vi "SysID Tracking.vi"(6 "PID Cluster":T4={"L1 to L4 PID Cluster"={"L1 PID Gains"={"Kp"=0.005, "Kd"=0.5, "Ki"=0.0005}, "L2 PID Gains"={"Kp"=0.01, "Kd"=1.0, "Ki"=0.005}, "L3 PID Gains"={"Kp"=0.05, "Kd"=1.0, "Ki"=0.0005}, "L4 PID Gains"={"Kp"=0.1, "Kd"=0.1, "Ki"=0.0005}}, "Stage PID Cluster"={"Stage Z PID"={"Kp"=0.0005, "Kd"=0.001, "Ki"=0.0}, "Stage Y PID"={"Kp"=0.0003, "Kd"=0.01, "Ki"=0.0}, "Stage X PID"={"Kp"=0.0003, "Kd"=0.01, "Ki"=0.0}}, "OCT Z PID Gains"={"Kp"=0.0003, "Kd"=0.0001, "Ki"=0.01}}, 7 "Input RY Signals":T1, 8 "error in":errorcluster, 9 "Offset Home 2 RCM":dbl[](array[numeric])=[0.0, 0.0, 0.0, 0.0], 10 "Prev Posit Cmd":T3={"Prev L1 to L4 Posit"=[-0.5319, -0.035669172703475985, -2.0566170657346783, 0.9099264705882353], "Prev Stage Posit"=[6.002553885707208, 5.996566124542428, 5.995469940427586], "Prev OCT Z Posit"=-0.0}, 11 "FPGA VI Reference In":refnum<k20>) -> (0 "error out":errorcluster, 2 "Last Posit Cmd":T2={"Last L1 to L4 Posit"=[0.0, 0.0, 0.0, 0.0], "Last Stage Posit"=[6.0, 6.0, 6.0], "Last OCT Z Posit"=0.0}, 3 "FPGA VI Reference Out":refnum<k20>, 5 "Output RY Signals":T1)   [LabVIEW 2016]
uses:
  <vilib>/Platform/TimedLoop/XDataNode/timing_clust.ctl
  <vilib>/Platform/TimedLoop/XDataNode/nitl_modes.ctl
  <vilib>/Platform/TimedLoop/XDataNode/wakeup.ctl
  Global Variables.vi
  <vilib>/Platform/TimedLoop/XDataNode/XDataNode.xnode
  <vilib>/Platform/TimedLoop/XDataNode/XDNodeRunTimeDep.lvlib
  Library/KevinLibraryAll/labview/KevLib01.lvlib
panel:
  out "In Servo Loop":bool
  out "Loading Finished":bool
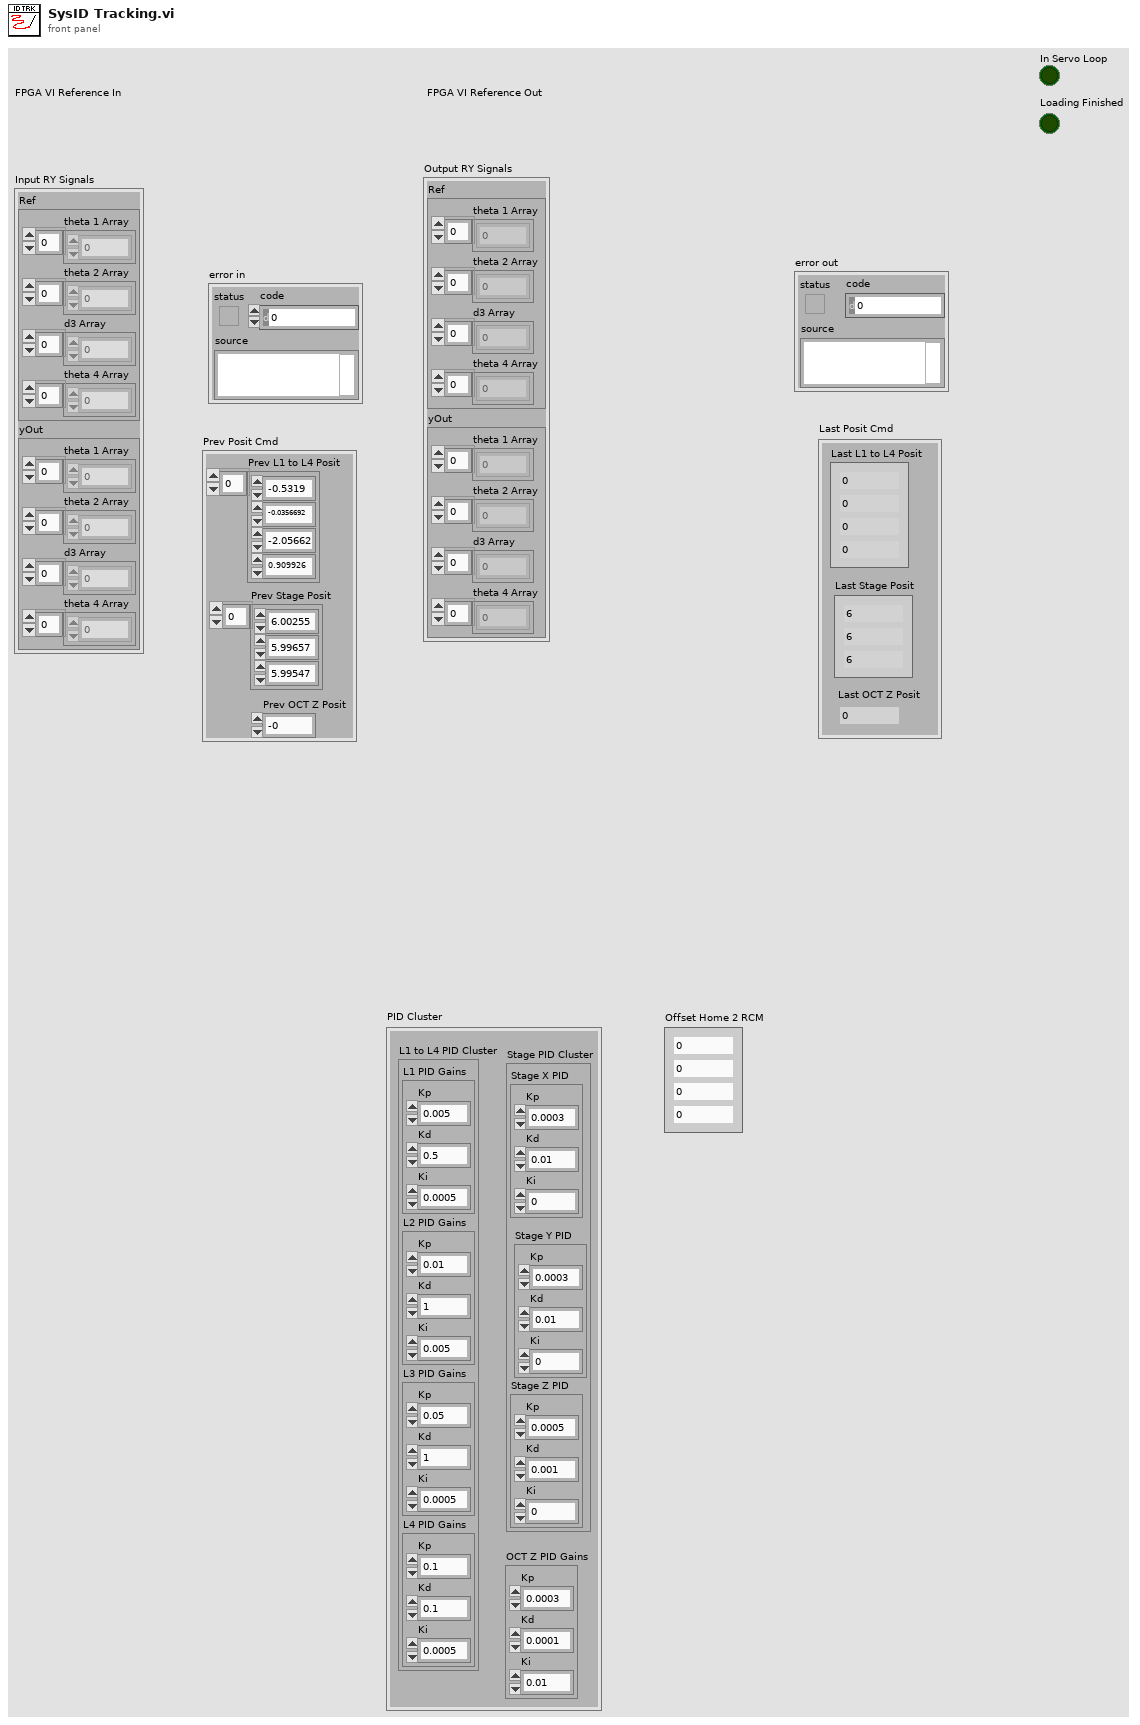
[diagram p1: front panel]
types:
  T1 = cluster{"Ref":cluster{"theta 1 Array":dbl[], "theta 2 Array":dbl[], "d3 Array":dbl[], "theta 4 Array":dbl[]}, "yOut":cluster{"theta 1 Array":dbl[], "theta 2 Array":dbl[], "d3 Array":dbl[], "theta 4 Array":dbl[]}}
  T2 = cluster{"Last L1 to L4 Posit":dbl[], "Last Stage Posit":dbl[], "Last OCT Z Posit":dbl}
  T3 = cluster{"Prev L1 to L4 Posit":dbl[], "Prev Stage Posit":dbl[], "Prev OCT Z Posit":dbl}
  T4 = cluster{"L1 to L4 PID Cluster":cluster{"L1 PID Gains":cluster{"Kp":dbl, "Kd":dbl, "Ki":dbl}, "L2 PID Gains":cluster{"Kp":dbl, "Kd":dbl, "Ki":dbl}, "L3 PID Gains":cluster{"Kp":dbl, "Kd":dbl, "Ki":dbl}, "L4 PID Gains":cluster{"Kp":dbl, "Kd":dbl, "Ki":dbl}}, "Stage PID Cluster":cluster{"Stage Z PID":cluster{"Kp":dbl, "Kd":dbl, "Ki":dbl}, "Stage Y PID":cluster{"Kp":dbl, "Kd":dbl, "Ki":dbl}, "Stage X PID":cluster{"Kp":dbl, "Kd":dbl, "Ki":dbl}}, "OCT Z PID Gains":cluster{"Kp":dbl, "Kd":dbl, "Ki":dbl}}
  T5 = cluster{"Stop Vacuum":bool, "Vacuum Force":i8, "Max Limit [mmHg]":dbl, "Slide in":i8, "Irrigation?":bool}
  T6 = typedef "XDNodeRunTimeDep.lvlib/timing_clust.ctl" = cluster{"Expected End [f-1]":u64, "Actual End [f-1]":u64, "Finished Late? [f-1]":bool, "Expected End [i-1]":u64, "Actual End [i-1]":u64, "Finished Late? [i-1]":bool, "Expected Start [i]":u64, "Actual Start [i]":u64, "Expected Start [f]":u64, "Actual Start [f]":u64, "Source Name":string, "Structure Name":string, "Period":i64, "Deadline":i64, "Offset":i64, "Start":i64, "Priority":i32, "Timeout":i32, "Mode":T7, "Wakeup Reason":T8, "Error":errorcluster, "Source Type":string, "Secondary Source Type":string, "Global End Time":u64, "Global Start Time":u64, "Frame Duration":u64, "Iteration Duration":u64, "Assigned CPU":i32, "I/O Scan Engine Mode":u32}
  T7 = typedef "XDNodeRunTimeDep.lvlib/nitl_modes.ctl" = enum32{"No Change", "Process missed periods, maintain original phase", "Discard missed periods, maintain original phase", "Process missed periods, ignore original phase", "Discard missed periods, ignore original phase"}
  T8 = typedef "XDNodeRunTimeDep.lvlib/wakeup.ctl" = enum32{"Normal", "Aborted", "Asynchronous wakeup", "Timing source error", "Timed loop error", "Timeout"}
  T9 = cluster{"L1 PID Gains":cluster{"Kp":dbl, "Kd":dbl, "Ki":dbl}, "L2 PID Gains":cluster{"Kp":dbl, "Kd":dbl, "Ki":dbl}, "L3 PID Gains":cluster{"Kp":dbl, "Kd":dbl, "Ki":dbl}, "L4 PID Gains":cluster{"Kp":dbl, "Kd":dbl, "Ki":dbl}}
  T10 = cluster{"Stage Z PID":cluster{"Kp":dbl, "Kd":dbl, "Ki":dbl}, "Stage Y PID":cluster{"Kp":dbl, "Kd":dbl, "Ki":dbl}, "Stage X PID":cluster{"Kp":dbl, "Kd":dbl, "Ki":dbl}}
  T11 = cluster{"Accurus button":bool[], "Accurus engaged?":bool, "Vacuum Force":i32, "Accurus Ch. A Vout":dbl, "Accurus Ch. B Vout":dbl, "Irrigation engaged?":bool}
  T12 = cluster{"theta 1 Array":dbl[], "theta 2 Array":dbl[], "d3 Array":dbl[], "theta 4 Array":dbl[]}
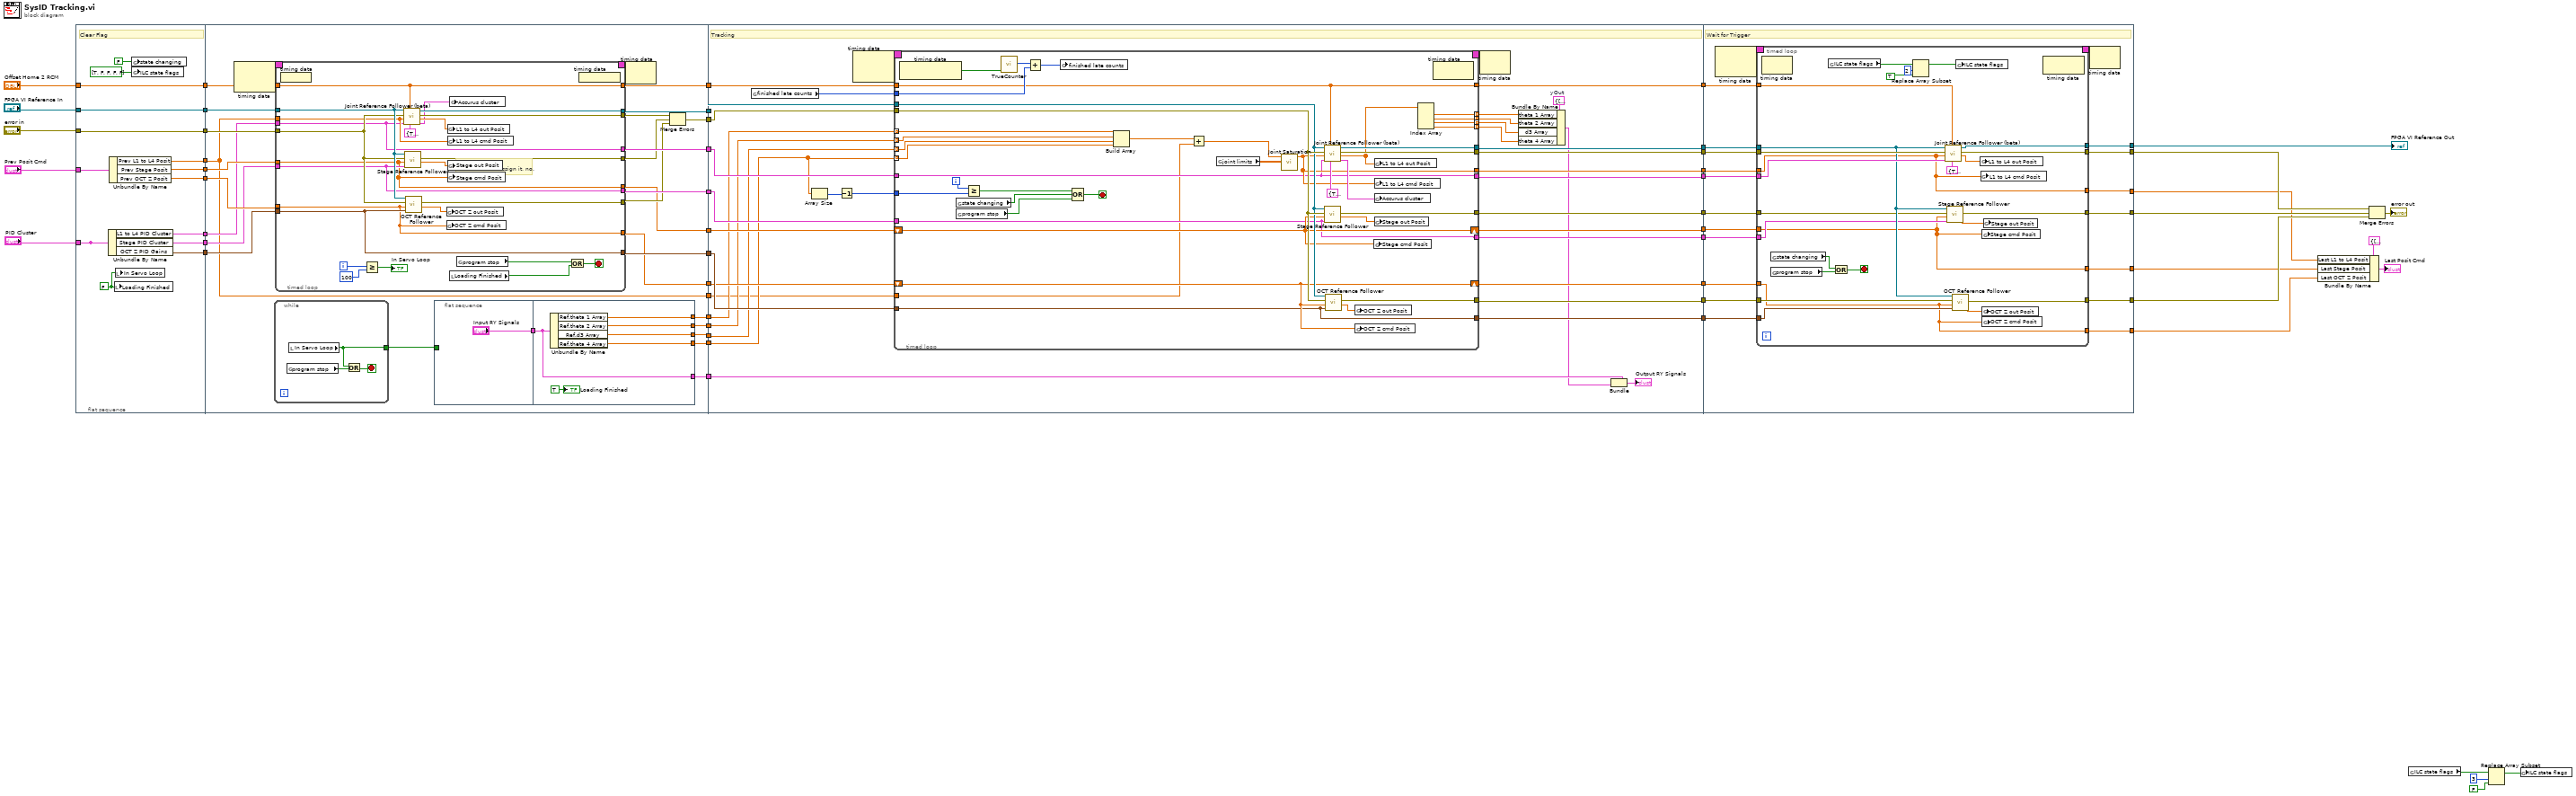
[diagram p0: block diagram]
diagram:
  n1 = flat-sequence {
    tunnel: [w67] -> w53
    tunnel: "FPGA VI Reference In" -> [w67]
    tunnel: "error in" -> [w66]
    tunnel: [w66] -> w51
    tunnel: "Prev Posit Cmd" -> [w65]
    tunnel: [w64] -> _
    tunnel: "PID Cluster" -> [w64]
    tunnel: [w63] -> w48
    tunnel: [w62] -> w47
    tunnel: [w61] -> w46
    tunnel: [w60] -> w45
    tunnel: [w59] -> w44
    tunnel: "Offset Home 2 RCM" -> [w59]
    tunnel: [w58] -> w39
    tunnel: [w56] -> w32
    tunnel: w53 -> [w96]
    tunnel: w51 -> [w95]
    tunnel: w48 -> [w94]
    tunnel: w47 -> [w93]
    tunnel: w46 -> [w92]
    tunnel: w45 -> [w91]
    tunnel: w44 -> [w90]
    tunnel: [w89] -> w42
    tunnel: [w88] -> w41
    tunnel: [w87] -> w40
    tunnel: w39 -> [w86]
    tunnel: [w85] -> w38
    tunnel: [w84] -> w37
    tunnel: [w83] -> w36
    tunnel: w32 -> [w68]
    tunnel: [w77] -> w31
    tunnel: [w76] -> w30
    tunnel: [w73] -> w25
    tunnel: [w72] -> w24
    tunnel: [w71] -> w23
    tunnel: [w70] -> w22
    tunnel: [w69] -> w21
    tunnel: [w68] -> w14
    tunnel: w42 -> [w169]
    tunnel: w41 -> [w155]
    tunnel: w40 -> [w168]
    tunnel: w38 -> [w166]
    tunnel: w37 -> [w165]
    tunnel: w36 -> [w164]
    tunnel: w31 -> [w157]
    tunnel: w30 -> [w156]
    tunnel: w25 -> [w140]
    tunnel: w24 -> [w151]
    tunnel: w23 -> [w150]
    tunnel: w22 -> [w149]
    tunnel: w21 -> [w148]
    tunnel: [w163] -> w13
    tunnel: [w162] -> w12
    tunnel: [w161] -> w11
    tunnel: [w160] -> w10
    tunnel: [w152] -> w9
    tunnel: [w159] -> w8
    tunnel: [w158] -> w7
    tunnel: [w142] -> w6
    tunnel: [w141] -> w5
    tunnel: [w139] -> w4
    tunnel: [w138] -> w3
    tunnel: w14 -> [w136]
    tunnel: w13 -> [w233]
    tunnel: w12 -> [w232]
    tunnel: w11 -> [w226]
    tunnel: w10 -> [w227]
    tunnel: w9 -> [w231]
    tunnel: w8 -> [w229]
    tunnel: w7 -> [w228]
    tunnel: w6 -> [w234]
    tunnel: w5 -> [w230]
    tunnel: w3 -> [w225]
    tunnel: w4 -> [w224]
    tunnel: [w223] -> w18
    tunnel: [w222] -> w19
    tunnel: [w221] -> w20
    tunnel: [w220] -> w1
    tunnel: [w219] -> w17
    tunnel: [w218] -> w16
    tunnel: [w217] -> w15
    frame #0 {
      w57 = FALSE ("Loading Finished")
      # "Clear Flag"
      n2 = Unbundle By Name(w64) -> ("L1 to L4 PID Cluster"=w60:T9, "Stage PID Cluster"=w58:T10, "OCT Z PID Gains"=w63:cluster{"Kp":dbl, "Kd":dbl, "Ki":dbl})
      n3 = Unbundle By Name(w65) -> ("Prev L1 to L4 Posit"=w56:dbl[], "Prev Stage Posit"=w62:dbl[], "Prev OCT Z Posit"=w61:dbl)
      n4 = local write "Loading Finished"(w57) -> ()
      n5 = local write "In Servo Loop"(w57) -> ()
      n6 = global write "Global Variables.vi" "state changing"(FALSE ("state changing")) -> ()
      n7 = global write "Global Variables.vi" "ILC state flags"(bool[] [TRUE, FALSE, FALSE, FALSE, FALSE]) -> ()
    }
    frame #1 {
      # "terminate loop\nwhen it. no. > assign it. no."
      n8 = node-c288() -> (w82:T6)  [unwired: 2 in]
      n9 = while {
        tunnel: [w97] -> w75
        stop <- w99 stop-if-true
        n10 = global read "Global Variables.vi" "program stop"() -> (w98:bool)
        n11 = local read "In Servo Loop"() -> (w97:bool)
        n12 = Or(x=w97, y=w98) -> (x .or. y?=w99:bool)
      }
      n13 = timed-loop {
        timing: w82 -> [_]
        timing-out: [_] -> w81
        tunnel: [w108] -> w77
        tunnel: [w107] -> w76
        tunnel: [w124] -> w89
        tunnel: [w123] -> w80
        tunnel: [w122] -> w79
        tunnel: [w121] -> w78
        tunnel: w96 -> [w120]
        tunnel: w95 -> [w119]
        tunnel: w94 -> [w116]
        tunnel: w68 -> [w118]
        tunnel: w93 -> [w108]
        tunnel: w92 -> [w107]
        tunnel: w91 -> [w114]
        tunnel: w90 -> [w117]
        tunnel: [w117] -> w88
        tunnel: w86 -> [w115]
        tunnel: [w116] -> w83
        tunnel: [w115] -> w84
        tunnel: [w114] -> w85
        i -> [w113]
        stop <- w130 stop-if-true
        n14 = node-c288 ("Output Node")() -> ()  [unwired: 1 in]
        n15 = Greater Or Equal?(x=w113, y=100) -> (x >= y?=→"In Servo Loop":bool)
        n16 = call "Joint Reference Follower (beta).vi"("Accurus Ctrl Cluster"=T5 {"Stop Vacuum"=TRUE, "Vacuum Force"=0, "Max Limit [mmHg]"=600.0, "Slide in"=0, "Irrigation?"=TRUE}, "Offset Home2RCM [deg/mm]"=w117, "PID Ctrl Cluster"=w114, "Ref Array [deg/mm]"=w118, "error in"=w119, "FPGA VI Reference In"=w120) -> ("Accurus Output Cluster"=w109:T11, "Output Posit Array [deg/mm]"=w127:dbl[], "error out"=w123:errorcluster, "FPGA VI Reference Out"=w124:refnum<k20>)  [unwired: 2 in]
        n17 = call "Stage Reference Follower.vi"("Stage PID Cluster"=w115, "Stage cmd Posit [mm]"=w108, "error in"=w119, "FPGA VI Reference In"=w120) -> ("Stage out Posit [mm]"=w126:dbl[], "error out"=w122:errorcluster)  [unwired: 5 in, 1 out]
        n18 = call "OCT Reference Follower.vi"("OCT Z PID Gains"=w116, "OCT  Z cmd Posit [mm]"=w107, "error in"=w119, "FPGA VI Reference In"=w120) -> ("OCT  Z out Posit [mm]"=w125:dbl, "error out"=w121:errorcluster)  [unwired: 5 in, 1 out]
        n19 = global write "Global Variables.vi" "OCT Z out Posit"(w125) -> ()
        n20 = global write "Global Variables.vi" "OCT Z cmd Posit"(w107) -> ()
        n21 = global write "Global Variables.vi" "L1 to L4 out Posit"(w127) -> ()
        n22 = global write "Global Variables.vi" "L1 to L4 cmd Posit"(w118) -> ()
        n23 = global write "Global Variables.vi" "Stage out Posit"(w126) -> ()
        n24 = global write "Global Variables.vi" "Stage cmd Posit"(w108) -> ()
        n25 = global write "Global Variables.vi" "Accurus cluster"(w109) -> ()
        n26 = local read "Loading Finished"() -> (w129:bool)
        n27 = global read "Global Variables.vi" "program stop"() -> (w128:bool)
        n28 = Or(x=w128, y=w129) -> (x .or. y?=w130:bool)
        n29 = node-c288() -> ()  [unwired: 1 out]
      }
      n30 = flat-sequence {
        tunnel: w75 -> [_]
        tunnel: ["Input RY Signals"] -> w74
        tunnel: w74 -> [w101]
        tunnel: [w105] -> w72
        tunnel: [w104] -> w71
        tunnel: [w103] -> w70
        tunnel: [w102] -> w69
        tunnel: [w101] -> w73
        frame #0 {
        }
        frame #1 {
          n31 = Unbundle By Name(w101) -> ("Ref.theta 1 Array"=w105:dbl[], "Ref.theta 2 Array"=w104:dbl[], "Ref.d3 Array"=w103:dbl[], "Ref.theta 4 Array"=w102:dbl[])
          "Loading Finished" <- TRUE ("Loading Finished")
        }
      }
      n32 = node-c288(w81) -> ()  [unwired: 1 out]
      n33 = Merge Errors(w80, w79, w78) -> (w87:errorcluster)
    }
    frame #2 {
      w147 = T12 {"theta 1 Array"=[], "theta 2 Array"=[], "d3 Array"=[], "theta 4 Array"=[]}  # yOut
      # "Tracking"
      n34 = global read "Global Variables.vi" "finished late counts"() -> (w167:u16)
      n35 = Array Size(array=w148) -> (size(s)=w154:i32)
      n36 = Decrement(x=w154) -> (x-1=w153:i32)
      n37 = node-c288() -> (w171:T6)  [unwired: 2 in]
      n38 = timed-loop {
        timing: w171 -> [_]
        timing-out: [_] -> w170
        tunnel: w151 -> [w189] mode=indexing
        tunnel: w150 -> [w188] mode=indexing
        tunnel: w149 -> [w187] mode=indexing
        tunnel: w169 -> [w209]
        tunnel: w155 -> [w178]
        tunnel: w168 -> [w210]
        tunnel: [w211] -> w163
        tunnel: w166 -> [w177]
        tunnel: w167 -> [w205]
        tunnel: w165 -> [w176]
        tunnel: w164 -> [w175]
        shift-right: [w202] -> w159
        shift-left: w157 -> [w202]
        shift-right: [w201] -> w158
        shift-left: w156 -> [w201]
        tunnel: [w200] -> w161
        tunnel: [w199] -> w160
        tunnel: [w198] -> w162
        tunnel: w153 -> [w195]
        tunnel: w148 -> [w186] mode=indexing
        tunnel: [w185] -> w152
        tunnel: [w182] -> w146 mode=indexing
        tunnel: [w181] -> w145 mode=indexing
        tunnel: [w180] -> w144 mode=indexing
        tunnel: [w179] -> w143 mode=indexing
        tunnel: [w178] -> w142
        tunnel: [w177] -> w141
        tunnel: [w176] -> w138
        tunnel: [w175] -> w139
        tunnel: w136 -> [w174]
        i -> [w190]
        stop <- w191 stop-if-true
        # "Hold Position if not Engaged"
        n39 = node-c288() -> (w208:bool)  [unwired: 1 in]
        n40 = global read "Global Variables.vi" "state changing"() -> (w193:bool)
        n41 = global read "Global Variables.vi" "program stop"() -> (w192:bool)
        n42 = Greater Or Equal?(x=w190, y=w195) -> (x >= y?=w194:bool)
        n43 = call "TrueCounter.vi"("True?"=w208) -> ("True Count"=w206:u16)  [unwired: 10 in]
        n44 = Add(x=w206, y=w205) -> (x+y=w207:u16)
        n45 = global write "Global Variables.vi" "finished late counts"(w207) -> ()
        n46 = Compound Arithmetic op=OR(w194, w193, w192) -> (w191:bool)
        n47 = Build Array(w189, w188, w187, w186) -> (w173:dbl[])
        n48 = Add(x=w173, y=w174) -> (x+y=w172:dbl[])
        n49 = global read "Global Variables.vi" "joint limits"() -> (w184:dbl[][])
        n50 = call "Joint Saturation.vi"("Joint Bounds [Deg/mm]"=w184, "Ref Array [Deg/mm]"=w172) -> ("Sat Ref Array [Deg/mm]"=w185:dbl[])  [unwired: 9 in]
        n51 = call "Joint Reference Follower (beta).vi"("Accurus Ctrl Cluster"=T5 {"Stop Vacuum"=TRUE, "Vacuum Force"=0, "Max Limit [mmHg]"=600.0, "Slide in"=0, "Irrigation?"=FALSE}, "Offset Home2RCM [deg/mm]"=w178, "PID Ctrl Cluster"=w177, "Ref Array [deg/mm]"=w185, "error in"=w210, "FPGA VI Reference In"=w209) -> ("Accurus Output Cluster"=w197:T11, "Output Posit Array [deg/mm]"=w183:dbl[], "error out"=w198:errorcluster, "FPGA VI Reference Out"=w211:refnum<k20>)  [unwired: 2 in]
        n52 = call "Stage Reference Follower.vi"("Stage PID Cluster"=w176, "Stage cmd Posit [mm]"=w202, "error in"=w210, "FPGA VI Reference In"=w209) -> ("Stage out Posit [mm]"=w204:dbl[], "error out"=w200:errorcluster)  [unwired: 5 in, 1 out]
        n53 = call "OCT Reference Follower.vi"("OCT Z PID Gains"=w175, "OCT  Z cmd Posit [mm]"=w201, "error in"=w210, "FPGA VI Reference In"=w209) -> ("OCT  Z out Posit [mm]"=w203:dbl, "error out"=w199:errorcluster)  [unwired: 5 in, 1 out]
        n54 = global write "Global Variables.vi" "OCT Z out Posit"(w203) -> ()
        n55 = global write "Global Variables.vi" "OCT Z cmd Posit"(w201) -> ()
        n56 = global write "Global Variables.vi" "Stage cmd Posit"(w202) -> ()
        n57 = global write "Global Variables.vi" "L1 to L4 out Posit"(w183) -> ()
        n58 = global write "Global Variables.vi" "L1 to L4 cmd Posit"(w185) -> ()
        n59 = global write "Global Variables.vi" "Accurus cluster"(w197) -> ()
        n60 = global write "Global Variables.vi" "Stage out Posit"(w204) -> ()
        n61 = Index Array(array=w183) -> (element #1=w182:dbl, element #2=w181:dbl, element #3=w180:dbl, element #4=w179:dbl)  [unwired: 4 in]
        n62 = node-c288() -> ()  [unwired: 1 in, 1 out]
      }
      n63 = node-c288(w170) -> ()  [unwired: 1 out]
      n64 = Bundle By Name(cluster=w147, "theta 1 Array"=w146, "theta 2 Array"=w145, "d3 Array"=w144, "theta 4 Array"=w143) -> (w137:T12)
      n65 = Bundle(cluster=w140, "yOut"=w137) -> (→"Output RY Signals":T1)  [unwired: 1 in]
    }
    frame #3 {
      # "Wait for Trigger"
      n66 = node-c288() -> (w236:T6)  [unwired: 2 in]
      n67 = timed-loop {
        timing: w236 -> [_]
        timing-out: [_] -> w235
        tunnel: w234 -> [w252]
        tunnel: w233 -> [w248]
        tunnel: w232 -> [w251]
        tunnel: w231 -> [w239]
        tunnel: w230 -> [w250]
        tunnel: w229 -> [w238]
        tunnel: w228 -> [w237]
        tunnel: w227 -> [w249]
        tunnel: w226 -> [w247]
        tunnel: w225 -> [w246]
        tunnel: w224 -> [w245]
        tunnel: [w243] -> w223
        tunnel: [w242] -> w222
        tunnel: [w241] -> w221
        tunnel: [w240] -> w220
        tunnel: [w239] -> w219
        tunnel: [w238] -> w218
        tunnel: [w237] -> w217
        stop <- w244 stop-if-true
        n68 = node-c288() -> ()  [unwired: 1 in, 1 out]
        n69 = global read "Global Variables.vi" "program stop"() -> (w258:bool)
        n70 = global read "Global Variables.vi" "state changing"() -> (w254:bool)
        n71 = global read "Global Variables.vi" "ILC state flags"() -> (w257:bool[])
        n72 = Or(x=w254, y=w258) -> (x .or. y?=w244:bool)
        n73 = Replace Array Subset(array=w257, new element=TRUE ("new element/subarray"), index=2) -> (w255:bool[])
        n74 = call "Joint Reference Follower (beta).vi"("Accurus Ctrl Cluster"=T5 {"Stop Vacuum"=TRUE, "Vacuum Force"=0, "Max Limit [mmHg]"=600.0, "Slide in"=0, "Irrigation?"=FALSE}, "Offset Home2RCM [deg/mm]"=w252, "PID Ctrl Cluster"=w250, "Ref Array [deg/mm]"=w239, "error in"=w251, "FPGA VI Reference In"=w248) -> ("Output Posit Array [deg/mm]"=w262:dbl[], "error out"=w243:errorcluster, "FPGA VI Reference Out"=w240:refnum<k20>)  [unwired: 2 in, 1 out]
        n75 = call "Stage Reference Follower.vi"("Stage PID Cluster"=w246, "Stage cmd Posit [mm]"=w238, "error in"=w247, "FPGA VI Reference In"=w248) -> ("Stage out Posit [mm]"=w261:dbl[], "error out"=w242:errorcluster)  [unwired: 5 in, 1 out]
        n76 = call "OCT Reference Follower.vi"("OCT Z PID Gains"=w245, "OCT  Z cmd Posit [mm]"=w237, "error in"=w249, "FPGA VI Reference In"=w248) -> ("OCT  Z out Posit [mm]"=w260:dbl, "error out"=w241:errorcluster)  [unwired: 5 in, 1 out]
        n77 = global write "Global Variables.vi" "ILC state flags"(w255) -> ()
        n78 = global write "Global Variables.vi" "L1 to L4 out Posit"(w262) -> ()
        n79 = global write "Global Variables.vi" "L1 to L4 cmd Posit"(w239) -> ()
        n80 = global write "Global Variables.vi" "OCT Z out Posit"(w260) -> ()
        n81 = global write "Global Variables.vi" "Stage cmd Posit"(w238) -> ()
        n82 = global write "Global Variables.vi" "OCT Z cmd Posit"(w237) -> ()
        n83 = global write "Global Variables.vi" "Stage out Posit"(w261) -> ()
        n84 = node-c288() -> ()  [unwired: 1 in, 1 out]
      }
      n85 = node-c288(w235) -> ()  [unwired: 1 out]
    }
  }
  n86 = Bundle By Name(cluster=T2 {"Last L1 to L4 Posit"=[0.0, 0.0, 0.0, 0.0], "Last Stage Posit"=[6.0, 6.0, 6.0], "Last OCT Z Posit"=0.0} ("Last Posit Cluster 2"), "Last L1 to L4 Posit"=w17, "Last Stage Posit"=w16, "Last OCT Z Posit"=w15) -> (→"Last Posit Cmd":T2)
  n87 = Merge Errors(w18, w19, w20) -> (→"error out":errorcluster)
  n88 = global read "Global Variables.vi" "ILC state flags"() -> (w27:bool[])
  n89 = Replace Array Subset(array=w27, new element=FALSE ("new element/subarray"), index=3) -> (w26:bool[])
  n90 = global write "Global Variables.vi" "ILC state flags"(w26) -> ()
  "FPGA VI Reference Out" <- w1
